vi "RotMoveScan.vi"(8 "error in (no error)":errorcluster, 11 "Microscope in":refnum<class "Microscope.lvclass">) -> (0 "error out":errorcluster, 3 "Microscope out":refnum<class "Microscope.lvclass">)   [LabVIEW 2012, in "Microscope.lvclass"]
uses:
  classes/Microscope.lvclass
  typedefs/Move Type.ctl
  classes/Microscope.lvclass/Microscope.ctl
  sub_vis/TriggererBoolean.vi
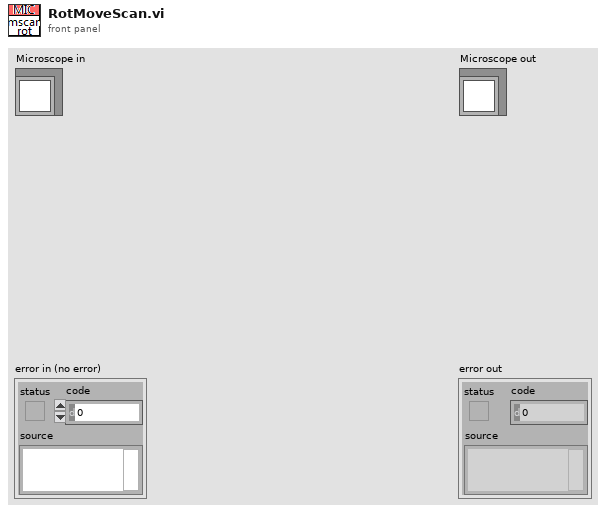
[diagram p1: front panel]
types:
  T1 = typedef "Move Type.ctl" = enum16{"None", "Continuous", "Discrete"}
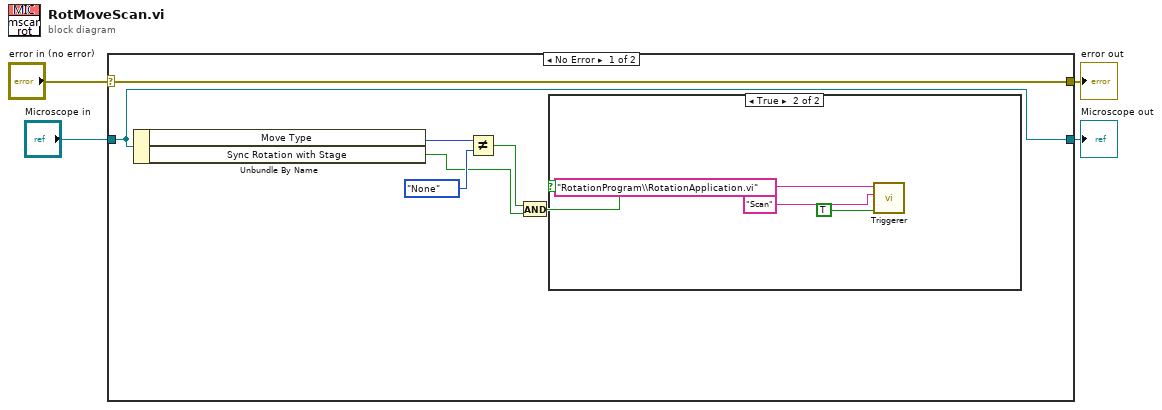
[diagram p0: block diagram]
diagram:
  n1 = case shown="No Error" "error in (no error)" {
    selector: "error in (no error)" -> [w11 w16]
    tunnel: [w11 w16] -> w3
    tunnel: [w8 w15] -> w1
    tunnel: "Microscope in" -> [w8 w15]
    frame No Error {
      n2 = Unbundle By Name(w8) -> ("Move Type"=w10:T1, "Sync Rotation with Stage"=w6:bool)
      n3 = Not Equal?(x=w10, y=Move_Type."None") -> (x != y?=w7:bool)
      n4 = And(x=w7, y=w6) -> (x .and. y?=w5:bool)
      n5 = case shown="True" w5 {
        frame False {
        }
        frame True {
          n6 = call-poly "Triggerer.vi"("Boolean"=TRUE, "Control Name"="Scan", "name or relative path"="RotationProgram\\RotationApplication.vi") -> ()  [unwired: 7 in, 2 out]
        }
      }
    }
    frame Error {
    }
  }
  "error out" <- w3
  "Microscope out" <- w1
